vi "E2E_EB_CalculateCrc (Hella).vi"(9 "Counter":u8, 11 "Data":u8[](array[numeric])) -> (3 "CrcValue":u8)   [LabVIEW 2013]
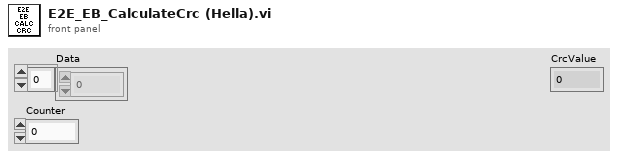
[diagram p1: front panel]
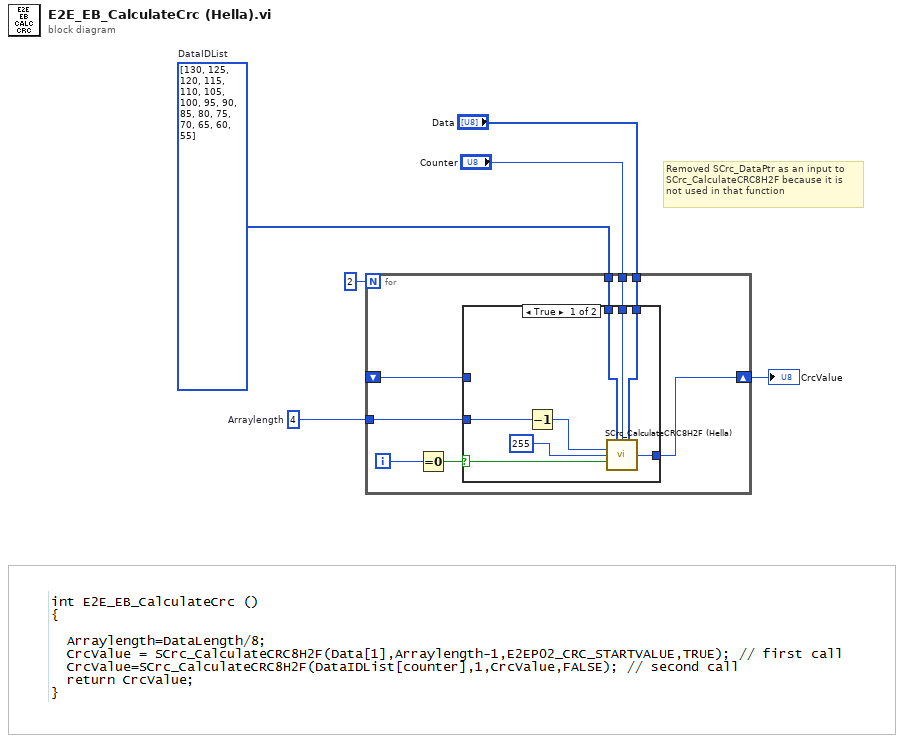
[diagram p0: block diagram]
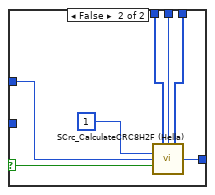
[diagram p2: hidden frame]
diagram:
  w5 = u8[] [130, 125, 120, 115, 110, 105, 100, 95, 90, 85, 80, 75, 70, 65, 60, 55]  # DataIDList
  w2 = u8 4  # Arraylength
  # "Removed SCrc_DataPtr as an input to\nSCrc_CalculateCRC8H2F because it is\nnot used in that function"
  n1 = for {
    N: 2 -> [_]
    tunnel: w5 -> [w12]
    tunnel: "Counter" -> [w11]
    tunnel: "Data" -> [w10]
    tunnel: w2 -> [w9]
    shift-right: [w8] -> w1
    shift-left: _ -> [w7]
    i -> [w14]
    n2 = Equal To 0?(x=w14) -> (x = 0?=w13:bool)
    n3 = case shown="True" w13 {
      selector: w13 -> [w22 w29]
      tunnel: [w21 w28] -> w8
      tunnel: w12 -> [w20 w26]
      tunnel: w11 -> [w19 w25]
      tunnel: w10 -> [w18 w27]
      tunnel: w9 -> [w17 _]
      tunnel: w7 -> [_ w23]
      frame True {
        n4 = Decrement(x=w17) -> (x-1=w16:u8)
        n5 = call "SCrc_CalculateCRC8H2F (Hella).vi"("DataIDList"=w20, "Counter"=w19, "Data"=w18, "SCrc_Length"=w16, "SCrc_StartValue8H2F IN"=u8 255, "SCrc_IsFirstCall"=w22) -> ("SCrc_StartValue8H2F OUT"=w21:u8)  [unwired: 9 in]
      }
      frame False {
        n6 = call "SCrc_CalculateCRC8H2F (Hella).vi"("DataIDList"=w26, "Counter"=w25, "Data"=w27, "SCrc_Length"=u8 1, "SCrc_StartValue8H2F IN"=w23, "SCrc_IsFirstCall"=w29) -> ("SCrc_StartValue8H2F OUT"=w28:u8)  [unwired: 9 in]
      }
    }
  }
  "CrcValue" <- w1
